vi "密码与账户校对.vi"(8 "密码路径":path, 9 "密码":string, 10 "账户路径":path, 11 "账户":string) -> (2 "x与y？":bool)   [LabVIEW 2018]
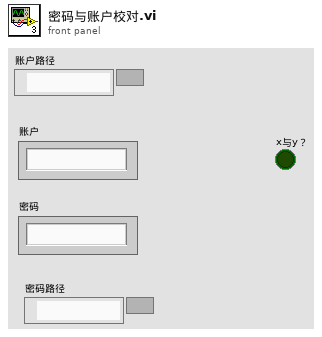
[diagram p1: front panel]
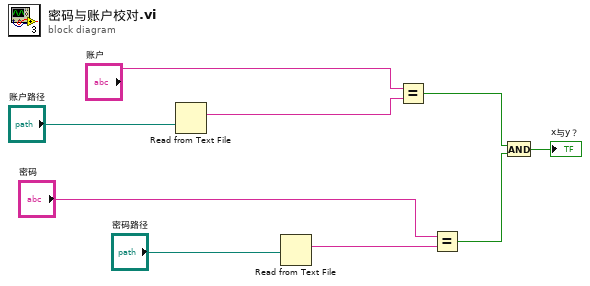
[diagram p0: block diagram]
diagram:
  n1 = Read from Text File(file (use dialog)="账户路径") -> (text=w8:string)  [unwired: 3 in, 3 out]
  n2 = Read from Text File(file (use dialog)="密码路径") -> (text=w5:string)  [unwired: 3 in, 3 out]
  n3 = Equal?(x="账户", y=w8) -> (x = y?=w3:bool)
  n4 = Equal?(x="密码", y=w5) -> (x = y?=w2:bool)
  n5 = And(x=w3, y=w2) -> (x .and. y?=→"x与y？":bool)
